vi "MainVI.vi"() -> ()   [LabVIEW 2014]
uses:
  <vilib>/addons/database/Connection.llb/DB Tools Open Connec (String).vi
  <vilib>/addons/database/Connection.llb/Conn Execute.vi
  <vilib>/addons/database/Recordset.llb/Rec Fetch Recordset Data (R).vi
  <vilib>/addons/database/Recordset.llb/Rec Destroy - Connection.vi
  <vilib>/addons/database/_DB Variant To Data/Database Variant To Data.xnode
  <vilib>/addons/database/NI_Database_API.lvlib
panel:
  out "error out":errorcluster
  in  "power spectrum 2":cluster{"f0":dbl, "df":dbl, "magnitude":dbl[]} {"magnitude" format="%.2p"; "f0" format="%0.2p"; "df" format="%0.2p"}
  in  "power spectrum":cluster{"f0":dbl, "df":dbl, "magnitude":dbl[]} {"magnitude" format="%.2p"; "f0" format="%0.2p"; "df" format="%0.2p"}
  in  "Exit":bool
  in  "Tab Control":enum32{"Log Data", " View Data"}(tab)
  out "Power Test":bool
  out "PowerResult":bool
  out "MicphoneResult":bool
  out "SPL @1Khz":dbl
  out "Micphone Test":bool
  out "TouchPanelResult":bool
  out "Touch panel Test":bool
  out "Earphone Test":bool
  in  "Start":bool
  out "THD":cluster{"f0":dbl, "df":dbl, "magnitude":dbl[]}(graph)
  out "UUT Serial #":string
  in  "Operator Name":string
  in  "CompactDB":bool
  in  "Order":enum32{"Ascend", "Descend"}(radio)
  in  "SortData":bool
  in  "GetData":bool
  out "Earphone THD":cluster{"f0":dbl, "df":dbl, "magnitude":dbl[]}(graph)
  in  "Records":i32(listbox)
  in  "Sort As":T1(ring)
  # "iPhone Test System"
  # "Step 1"
  # "Step 2"
  # "Step 3"
  # "High Limit: 65dB"
  # "dB"
  # "Low Limit: 55dB"
  # "Step 4"
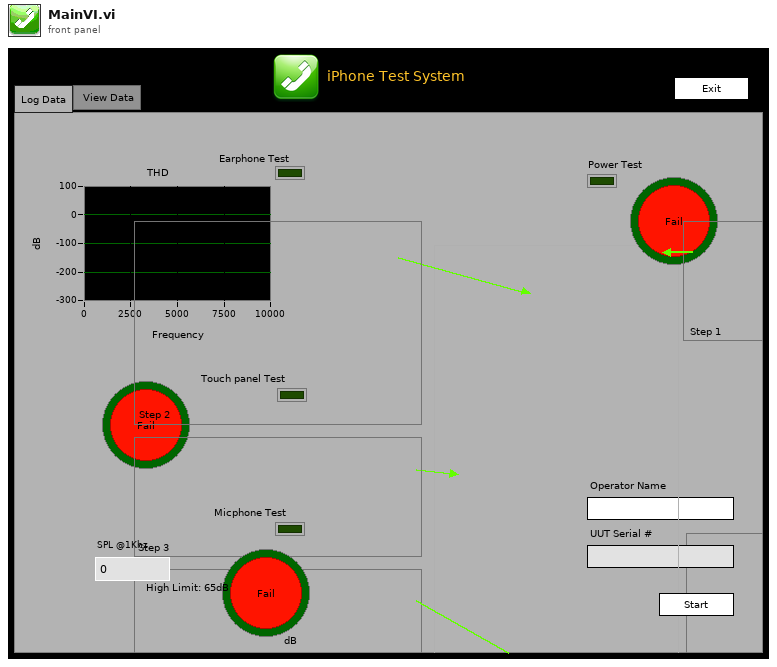
[diagram p1: front panel]
types:
  T1 = enum16{"Date/Time", "Operator", "UUT Serial", "MicphoneSPL"}
  T2 = cluster{string, "Operator Name":string, "UUT Serial #":string, "PowerResult":bool, "THD":cluster{"f0":dbl, "df":dbl, "magnitude":dbl[]}, "TouchPanelResult":bool, "MicPass?":bool, "SPL":dbl}
  T3 = typedef "NI_Database_API.lvlib/Conn ObjectReference.ctl" = refnum<k1>
  T4 = typedef "NI_Database_API.lvlib/Rec ObjectReference.ctl" = refnum<k1>
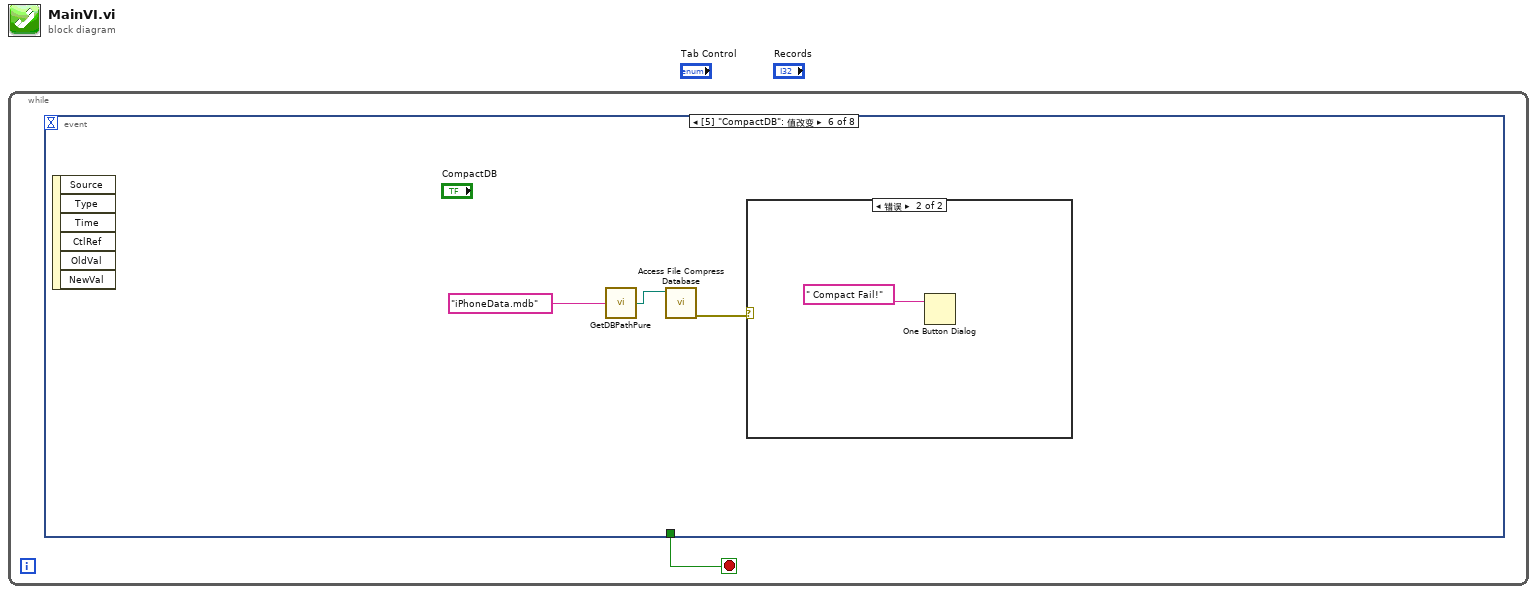
[diagram p0: block diagram]
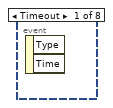
[diagram p2: hidden frame]
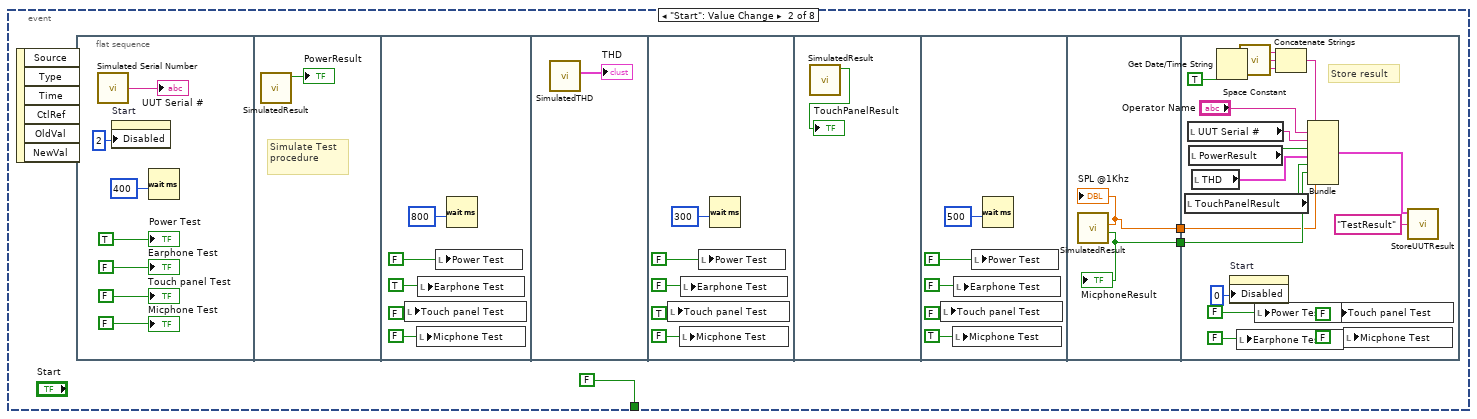
[diagram p3: hidden frame]
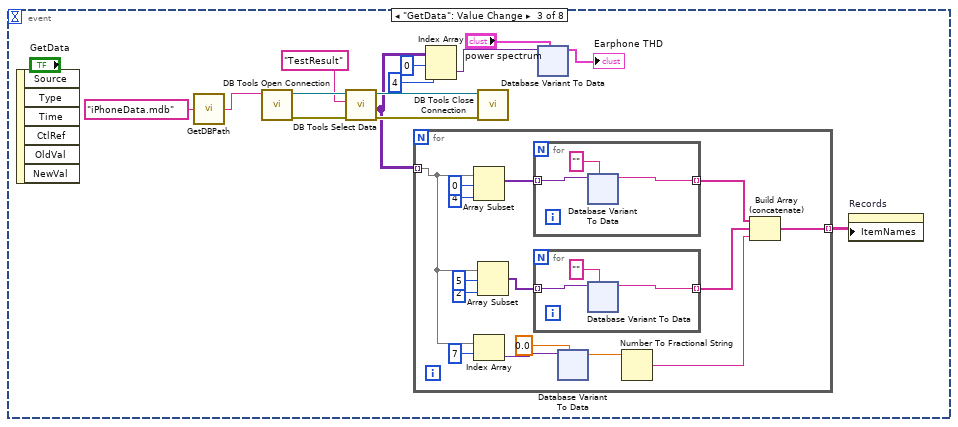
[diagram p4: hidden frame]
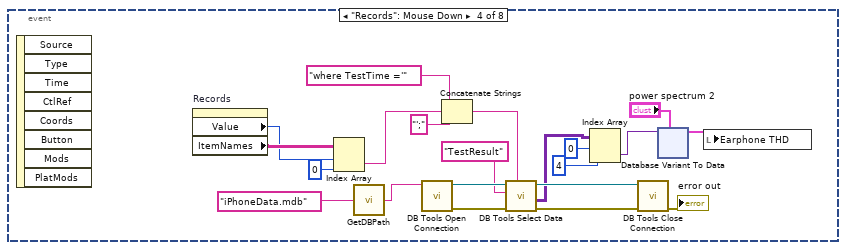
[diagram p5: hidden frame]
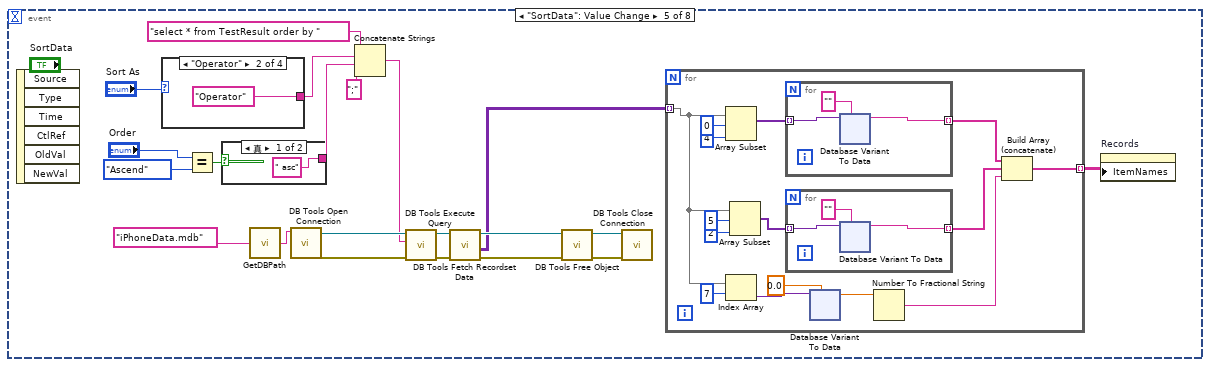
[diagram p6: hidden frame]
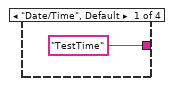
[diagram p7: hidden frame]
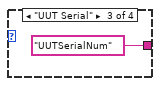
[diagram p8: hidden frame]
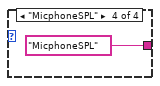
[diagram p9: hidden frame]
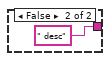
[diagram p10: hidden frame]
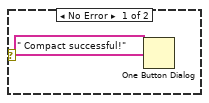
[diagram p11: hidden frame]
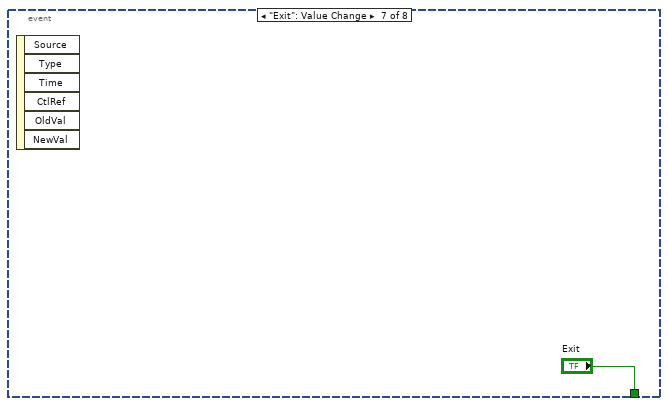
[diagram p12: hidden frame]
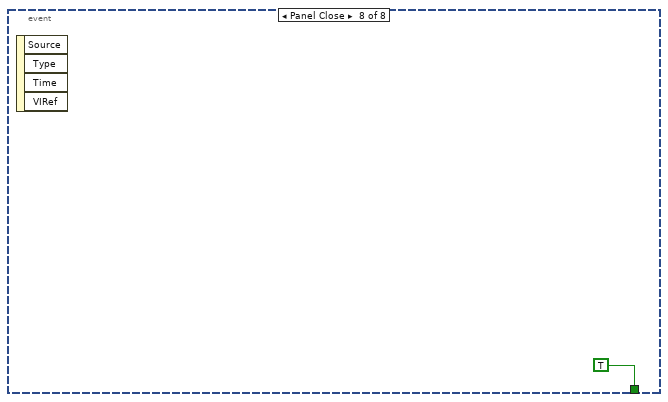
[diagram p13: hidden frame]
diagram:
  n1 = while {
    stop <- w1 stop-if-true
    n2 = event shown="[5] \"CompactDB\": 值改变" {
      selector: _ -> [_ _ _ _ _ _ _ _]
      dyn-events: _ -> [_ _ _ _ _ _ _ _]
      timeout: _ -> [_ _ _ _ _ _ _ _]
      tunnel: [_ FALSE _ _ _ _ "Exit" TRUE] -> w1
      event Timeout {
        n3 = event-data() -> ()  [unwired: 1 in, 2 out]
      }
      event "Start": Value Change {
        n4 = event-data() -> ()  [unwired: 1 in, 6 out]
        n5 = flat-sequence {
          tunnel: [w31] -> w3
          tunnel: [w30] -> w2
          tunnel: w3 -> [w39]
          tunnel: w2 -> [w38]
          frame #0 {
            n6 = call "Simulated Serial Number.vi"() -> ("UUT Serial #"=→"UUT Serial #":string)
            n7 = property on="Start" class="Bool"("Disabled"=u8 2) -> ()  [unwired: 2 in, 2 out]
            n8 = Wait (ms)(milliseconds to wait=u32 400) -> ()  [unwired: 1 out]
            "Power Test" <- TRUE
            "Earphone Test" <- FALSE
            "Touch panel Test" <- FALSE
            "Micphone Test" <- FALSE
          }
          frame #1 {
            # "Simulate Test\nprocedure"
            n9 = call "SimulatedResult.vi"() -> ("Pass?"=→"PowerResult":bool)  [unwired: 9 in, 2 out]
          }
          frame #2 {
            n10 = local write "Touch panel Test"(FALSE) -> ()
            n11 = local write "Micphone Test"(FALSE) -> ()
            n12 = local write "Earphone Test"(TRUE) -> ()
            n13 = local write "Power Test"(FALSE) -> ()
            n14 = Wait (ms)(milliseconds to wait=u32 800) -> ()  [unwired: 1 out]
          }
          frame #3 {
            n15 = call "SimulatedTHD.vi"() -> ("THD"=→"THD":cluster{"f0":dbl, "df":dbl, "magnitude":dbl[]})  [unwired: 10 in, 1 out]
          }
          frame #4 {
            n16 = local write "Touch panel Test"(TRUE) -> ()
            n17 = local write "Micphone Test"(FALSE) -> ()
            n18 = local write "Earphone Test"(FALSE) -> ()
            n19 = local write "Power Test"(FALSE) -> ()
            n20 = Wait (ms)(milliseconds to wait=u32 300) -> ()  [unwired: 1 out]
          }
          frame #5 {
            n21 = call "SimulatedResult.vi"() -> ("Pass?"=→"TouchPanelResult":bool)  [unwired: 9 in, 2 out]
          }
          frame #6 {
            n22 = local write "Touch panel Test"(FALSE) -> ()
            n23 = local write "Micphone Test"(TRUE) -> ()
            n24 = local write "Earphone Test"(FALSE) -> ()
            n25 = local write "Power Test"(FALSE) -> ()
            n26 = Wait (ms)(milliseconds to wait=u32 500) -> ()  [unwired: 1 out]
          }
          frame #7 {
            n27 = call "SimulatedResult.vi"() -> ("MicPass?"=w31:bool, "SPL"=w30:dbl)  [unwired: 9 in, 1 out]
            "SPL @1Khz" <- w30
            "MicphoneResult" <- w31
          }
          frame #8 {
            # "Store result"
            n28 = local read "TouchPanelResult"() -> (w40:bool)
            n29 = local read "UUT Serial #"() -> (w43:string)
            n30 = local read "PowerResult"() -> (w42:bool)
            n31 = local read "THD"() -> (w41:cluster{"f0":dbl, "df":dbl, "magnitude":dbl[]})
            n32 = Get Date/Time String(want seconds? (F)=TRUE) -> (date string=w35:string, time string=w33:string)  [unwired: 2 in]
            n33 = property on="Start" class="Bool"("Disabled"=u8 0) -> ()  [unwired: 2 in, 2 out]
            n34 = local write "Earphone Test"(FALSE) -> ()
            n35 = call <vilib>:"Space Constant.vi"() -> ("String"=w34:string)
            n36 = local write "Power Test"(FALSE) -> ()
            n37 = Concatenate Strings(w35, w34, w33) -> (w32:string)
            n38 = Bundle(w32, "Operator Name"="Operator Name", "UUT Serial #"=w43, "PowerResult"=w42, "THD"=w41, "TouchPanelResult"=w40, "MicPass?"=w39, "SPL"=w38) -> (w37:T2)  [unwired: 1 in]
            n39 = local write "Touch panel Test"(FALSE) -> ()
            n40 = local write "Micphone Test"(FALSE) -> ()
            n41 = call "StoreUUTResult.vi"("Table name"="TestResult", "Result"=w37) -> ()  [unwired: 9 in, 1 out]
          }
        }
      }
      event "GetData": Value Change {
        n42 = event-data() -> ()  [unwired: 1 in, 6 out]
        n43 = call "GetDBPath.vi"("Filename"="iPhoneData.mdb") -> ("Connection"=w63:string)
        n44 = call-poly <vilib>:"DB Tools Open Connection.vi"("connection information"=w63) -> ("error out"=w60:errorcluster, "connection reference"=w62:T3)  [unwired: 7 in]
        n45 = call <vilib>:"DB Tools Select Data.vi"("error in (no error)"=w60, "table"="TestResult", "connection reference"=w62) -> ("error out"=w58:errorcluster, "data"=w57:variant[][], "connection reference out"=w59:T3)  [unwired: 3 in]
        n46 = for {
          tunnel: w57 -> [w108] mode=indexing
          tunnel: [w100] -> w51 mode=indexing
          n47 = Array Subset(array=w108, index=0, length=4) -> (w112:variant[])
          n48 = Index Array(array=w108, index=7) -> (element=w106:variant)
          n49 = Array Subset(array=w108, index=5, length=2) -> (w109:variant[])
          n50 = for {
            tunnel: w112 -> [w184] mode=indexing
            tunnel: [w182] -> w101 mode=indexing
            n51 = xnode "Database Variant To Data"("database variant"=w184, "type"="") -> ("data"=w182:string)  [unwired: 1 in, 1 out]
          }
          n52 = for {
            tunnel: w109 -> [w149] mode=indexing
            tunnel: [w147] -> w102 mode=indexing
            n53 = xnode "Database Variant To Data"("database variant"=w149, "type"="") -> ("data"=w147:string)  [unwired: 1 in, 1 out]
          }
          n54 = xnode "Database Variant To Data"("database variant"=w106, "type"=0.0 ("number (0 to 1)")) -> ("data"=w104:dbl)  [unwired: 1 in, 1 out]
          n55 = Number To Fractional String(number=w104) -> (F-format string=w103:string)  [unwired: 3 in]
          n56 = Build Array (concatenate)(w101, w102, w103) -> (w100:string[])
        }
        n57 = Index Array(array=w57, index (row)=0, index (col)=4 ("disabled index (col)")) -> (element=w54:variant)
        n58 = call <vilib>:"DB Tools Close Connection.vi"("error in (no error)"=w58, "connection reference"=w59) -> ()  [unwired: 5 in, 1 out]
        n59 = xnode "Database Variant To Data"("database variant"=w54, "type"="power spectrum") -> ("data"=→"Earphone THD":cluster{"f0":dbl, "df":dbl, "magnitude":dbl[]})  [unwired: 1 in, 1 out]
        n60 = property on="Records" class="MCListbox (严格)"("ItemNames"=w51) -> ()  [unwired: 2 in, 2 out]
      }
      event "Records": Mouse Down {
        n61 = event-data() -> ()  [unwired: 1 in, 8 out]
        n62 = property on="Records" class="MCListbox (严格)"() -> ("Value"=w236:i32, "ItemNames"=w237:string[][])  [unwired: 2 in, 2 out]
        n63 = Index Array(array=w237, index (row)=w236, index (col)=0 ("disabled index (col)")) -> (element=w217:string)
        n64 = call "GetDBPath.vi"("Filename"="iPhoneData.mdb") -> ("Connection"=w233:string)
        n65 = call-poly <vilib>:"DB Tools Open Connection.vi"("connection information"=w233) -> ("error out"=w230:errorcluster, "connection reference"=w232:T3)  [unwired: 7 in]
        n66 = Concatenate Strings("where TestTime ='" ("string"), w217, "';" ("string")) -> (w226:string)
        n67 = call <vilib>:"DB Tools Select Data.vi"("condition"=w226, "error in (no error)"=w230, "table"="TestResult", "connection reference"=w232) -> ("error out"=w228:errorcluster, "data"=w223:variant[][], "connection reference out"=w229:T3)  [unwired: 2 in]
        n68 = Index Array(array=w223, index (row)=0, index (col)=4 ("disabled index (col)")) -> (element=w220:variant)
        n69 = call <vilib>:"DB Tools Close Connection.vi"("error in (no error)"=w228, "connection reference"=w229) -> ("error out"=→"error out":errorcluster)  [unwired: 5 in]
        n70 = xnode "Database Variant To Data"("database variant"=w220, "type"="power spectrum 2") -> ("data"=w218:cluster{"f0":dbl, "df":dbl, "magnitude":dbl[]})  [unwired: 1 in, 1 out]
        n71 = local write "Earphone THD"(w218) -> ()
      }
      event "SortData": Value Change {
        n72 = event-data() -> ()  [unwired: 1 in, 6 out]
        n73 = case shown="\"Operator\"" "Sort As" {
          tunnel: ["TestTime" "Operator" "UUTSerialNum" "MicphoneSPL"] -> w273
          frame "Date/Time", Default {
          }
          frame "Operator" {
          }
          frame "UUT Serial" {
          }
          frame "MicphoneSPL" {
          }
        }
        n74 = Equal?(x="Order", y=enum32{"Ascend", "Descend"}."Ascend" ("Order")) -> (x = y?=w291:bool)
        n75 = case shown="真" w291 {
          tunnel: [" asc" ("Substring") " desc" ("Substring")] -> w289
          frame True {
          }
          frame False {
          }
        }
        n76 = call "GetDBPath.vi"("Filename"="iPhoneData.mdb") -> ("Connection"=w287:string)
        n77 = call-poly <vilib>:"DB Tools Open Connection.vi"("connection information"=w287) -> ("error out"=w280:errorcluster, "connection reference"=w279:T3)  [unwired: 7 in]
        n78 = Concatenate Strings("select * from TestResult order by " ("SQL query"), w273, w289, ";" ("Substring")) -> (w278:string)
        n79 = call-poly <vilib>:"DB Tools Execute Query.vi"("error in (no error)"=w280, "SQL query"=w278, "connection reference"=w279) -> ("error out"=w282:errorcluster, "recordset reference"=w281:T4)  [unwired: 5 in]
        n80 = call-poly <vilib>:"DB Tools Fetch Recordset Data.vi"("error in (no error)"=w282, "recordset reference"=w281) -> ("error out"=w283:errorcluster, "recordset data"=w275:variant[][], "recordset reference out"=w284:T4)  [unwired: 3 in]
        n81 = call-poly <vilib>:"DB Tools Free Object.vi"("error in (no error)"=w283, "recordset reference"=w284) -> ("error out"=w286:errorcluster, "connection reference"=w285:T3)  [unwired: 8 in]
        n82 = call <vilib>:"DB Tools Close Connection.vi"("error in (no error)"=w286, "connection reference"=w285) -> ()  [unwired: 5 in, 1 out]
        n83 = for {
          tunnel: w275 -> [w306] mode=indexing
          tunnel: [w298] -> w276 mode=indexing
          n84 = Array Subset(array=w306, index=0, length=4) -> (w310:variant[])
          n85 = Index Array(array=w306, index=7) -> (element=w304:variant)
          n86 = Array Subset(array=w306, index=5, length=2) -> (w307:variant[])
          n87 = for {
            tunnel: w310 -> [w382] mode=indexing
            tunnel: [w380] -> w299 mode=indexing
            n88 = xnode "Database Variant To Data"("database variant"=w382, "type"="") -> ("data"=w380:string)  [unwired: 1 in, 1 out]
          }
          n89 = for {
            tunnel: w307 -> [w347] mode=indexing
            tunnel: [w345] -> w300 mode=indexing
            n90 = xnode "Database Variant To Data"("database variant"=w347, "type"="") -> ("data"=w345:string)  [unwired: 1 in, 1 out]
          }
          n91 = xnode "Database Variant To Data"("database variant"=w304, "type"=0.0 ("number (0 to 1)")) -> ("data"=w302:dbl)  [unwired: 1 in, 1 out]
          n92 = Number To Fractional String(number=w302) -> (F-format string=w301:string)  [unwired: 3 in]
          n93 = Build Array (concatenate)(w299, w300, w301) -> (w298:string[])
        }
        n94 = property on="Records" class="MCListbox (严格)"("ItemNames"=w276) -> ()  [unwired: 2 in, 2 out]
      }
      event "CompactDB": Value Change {
        n95 = event-data() -> ()  [unwired: 1 in, 6 out]
        n96 = call "GetDBPathPure.vi"("Filename"="iPhoneData.mdb") -> ("Connection"=w418:path)
        n97 = call "Access File Compress Database.vi"("Access File Path"=w418) -> ("error out"=w417:errorcluster)  [unwired: 10 in]
        n98 = case shown="错误" w417 {
          frame No Error {
            n99 = One Button Dialog(message=" Compact successful!") -> ()  [unwired: 1 in, 1 out]
          }
          frame Error {
            n100 = One Button Dialog(message=" Compact Fail!") -> ()  [unwired: 1 in, 1 out]
          }
        }
      }
      event "Exit": Value Change {
        n101 = event-data() -> ()  [unwired: 1 in, 6 out]
      }
      event Panel Close {
        n102 = event-data() -> ()  [unwired: 1 in, 4 out]
      }
    }
  }
